vi "Get_No_Top_Level_Message.vi"(11 "Build in":refnum<class "AB_InteropAssembly.lvclass">) -> (2 "No top level VI":string, 3 "Build out":refnum<class "AB_InteropAssembly.lvclass">)   [LabVIEW 2020, in "AB_InteropAssembly.lvclass"]
uses:
  <vilib>/AppBuilder/AB_Classes/InteropAssembly/AB_InteropAssembly.lvclass
  <vilib>/AppBuilder/AB_Classes/InteropAssembly/AB_InteropAssembly.lvclass/AB_InteropAssembly.ctl
  <resource>/Framework/Providers/Common/provcom_StringGlobals.vi
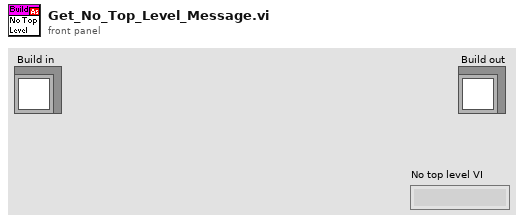
[diagram p1: front panel]
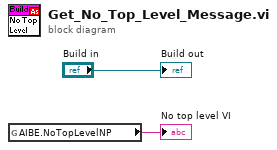
[diagram p0: block diagram]
diagram:
  n1 = global read "provcom_StringGlobals.vi" "AIBE.NoTopLevelNP"() -> (→"No top level VI":string)
  "Build out" <- "Build in"
